vi "Make path.vi"(8 "error in (no error)":errorcluster, 10 "File type":T1, 11 "Tomo in":refnum<class "Tomo.lvclass">) -> (0 "error out":errorcluster, 2 "path":path, 3 "Tomo out":refnum<class "Tomo.lvclass">)   [LabVIEW 2012, in "Tomo.lvclass"]
uses:
  Tomo.lvclass
  file type.ctl
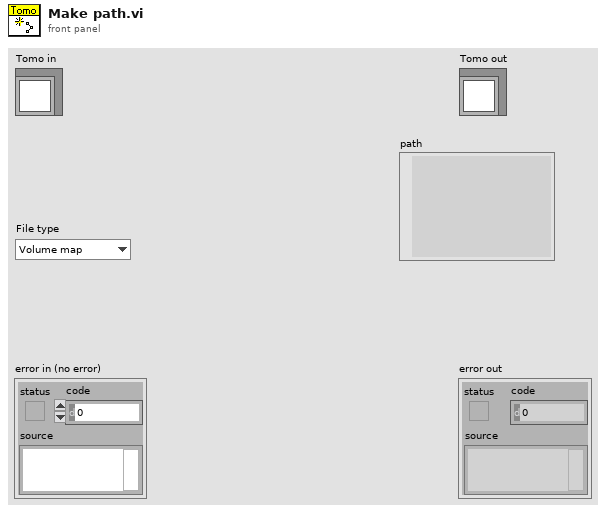
[diagram p1: front panel]
types:
  T1 = typedef "Tomo.lvclass/file type.ctl" = enum16{"Volume map", "Completed stacks"}
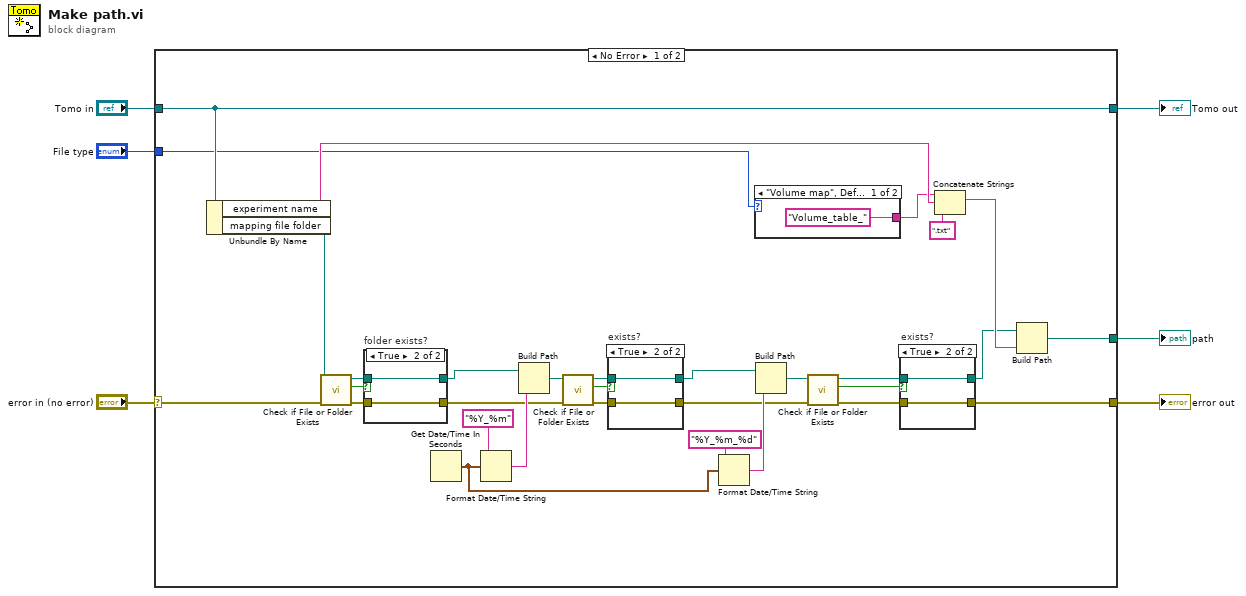
[diagram p0: block diagram]
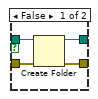
[diagram p2: hidden frame]
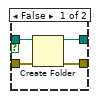
[diagram p3: hidden frame]
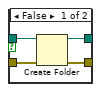
[diagram p4: hidden frame]
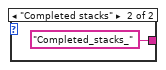
[diagram p5: hidden frame]
diagram:
  n1 = case shown="No Error" "error in (no error)" {
    selector: "error in (no error)" -> [w28 w59]
    tunnel: [w7 w59] -> w5
    tunnel: [w36 w58] -> w3
    tunnel: "Tomo in" -> [w36 w58]
    tunnel: [w26 _] -> w2
    tunnel: "File type" -> [w34 _]
    frame No Error {
      n2 = Unbundle By Name(w36) -> ("experiment name"=w35:string, "mapping file folder"=w32:path)
      n3 = call <vilib>:"Check if File or Folder Exists.vi"("error in (no error)"=w28, "path"=w32) -> ("error out"=w29:errorcluster, "file or folder exists?"=w30:bool, "dup path"=w31:path)  [unwired: 7 in]
      n4 = case "folder exists?" shown="True" w30 {
        tunnel: w31 -> [w53 w55]
        tunnel: w29 -> [w52 w54]
        tunnel: [w51 w54] -> w10
        tunnel: [w50 w55] -> w9
        frame False {
          n5 = Create Folder(path (use dialog)=w53, error in=w52) -> (created path=w50:path, error out=w51:errorcluster)  [unwired: 1 in, 1 out]
        }
        frame True {
        }
      }
      n6 = Get Date/Time In Seconds() -> (seconds since 1Jan1904=w11:timestamp)
      n7 = Format Date/Time String(time format string (%c)="%Y_%m", seconds (now)=w11) -> (date/time string=w25:string)  [unwired: 1 in]
      n8 = Build Path(base path=w9, name or relative path=w25) -> (appended path=w23:path)
      n9 = call <vilib>:"Check if File or Folder Exists.vi"("error in (no error)"=w10, "path"=w23) -> ("error out"=w20:errorcluster, "file or folder exists?"=w22:bool, "dup path"=w21:path)  [unwired: 7 in]
      n10 = case "exists?" shown="True" w22 {
        tunnel: w21 -> [w46 w48]
        tunnel: w20 -> [w47 w49]
        tunnel: [w45 w48] -> w12
        tunnel: [w44 w49] -> w13
        frame False {
          n11 = Create Folder(path (use dialog)=w46, error in=w47) -> (created path=w45:path, error out=w44:errorcluster)  [unwired: 1 in, 1 out]
        }
        frame True {
        }
      }
      n12 = Format Date/Time String(time format string (%c)="%Y_%m_%d", seconds (now)=w11) -> (date/time string=w15:string)  [unwired: 1 in]
      n13 = case shown="\"Volume map\", Default" w34 {
        tunnel: ["Volume_table_" ("string") "Completed_stacks_" ("string")] -> w33
        frame "Volume map", Default {
        }
        frame "Completed stacks" {
        }
      }
      n14 = Build Path(base path=w12, name or relative path=w15) -> (appended path=w19:path)
      n15 = call <vilib>:"Check if File or Folder Exists.vi"("error in (no error)"=w13, "path"=w19) -> ("error out"=w16:errorcluster, "file or folder exists?"=w18:bool, "dup path"=w17:path)  [unwired: 7 in]
      n16 = case "exists?" shown="True" w18 {
        tunnel: w17 -> [w40 w42]
        tunnel: w16 -> [w41 w43]
        tunnel: [w39 w42] -> w8
        tunnel: [w38 w43] -> w7
        frame False {
          n17 = Create Folder(path (use dialog)=w40, error in=w41) -> (created path=w39:path, error out=w38:errorcluster)  [unwired: 1 in, 1 out]
        }
        frame True {
        }
      }
      n18 = Concatenate Strings(w33, w35, ".txt" ("string")) -> (w27:string)
      n19 = Build Path(base path=w8, name or relative path=w27) -> (appended path=w26:path)
    }
    frame Error {
    }
  }
  "error out" <- w5
  "Tomo out" <- w3
  "path" <- w2
